vi "VI Reference Includes.vi"   [LabVIEW 2013, in "Engine Runtime Interface.lvclass"]
uses:
  Engine Runtime Interface.lvclass
  Engine Configuration/add and map fixed channel mapping.vi
  Engine Configuration/rename channel in mapping.vi
  Engine Configuration/apply mapping changes.vi
  Engine Configuration/delete mapping by channel.vi
  Engine Configuration/add mapping.vi
  Engine Configuration/apply tag changes.vi
  Engine Configuration/locate tag by name.vi
  Engine Configuration/delete tag.vi
  Engine Configuration/change tag metadata.vi
  Engine Configuration/change tag raw default value.vi
  Engine Configuration/change tag type.vi
  Engine Configuration/rename tag.vi
  Engine Configuration/add tag.vi
  Engine Configuration/Mappings.ctl
  Engine Configuration/Module Mappings.ctl
  Engine Configuration/Tag Info.ctl
  Engine Configuration/instance count allowed.vi
  Engine Configuration/get runtime class name.vi
  Engine Configuration/Get Supported Targets.vi
  Engine Configuration/filter tags by writer.vi
  Engine Configuration/filter tags by owner.vi
  Engine Configuration/filter tags by readers.vi
  Engine Configuration/filter tags available for mapping to channel.vi
  Engine Configuration/get full tag list.vi
  Engine Configuration/find tag mapped to channel.vi
  Engine Configuration/engine version.vi
  Engine Configuration/from string.vi
  Engine Configuration/to string.vi
  Engine Configuration/validate configuration.vi
  Get Unmapped Outputs.vi
  Get Mapping By Type.vi
  Find Tag From Channel Name.vi
  Find Components Mapping From Component or Channel Name.vi
  Create New Tags and Mappings.vi
  Append New Mappings.vi
  Create Tag Channel Pair.vi
  Execution States.ctl
  Open.vi
  Initialize.vi
  Start.vi
  Set Safe State.vi
  Pause.vi
  Get State.vi
  Stop.vi
  Close.vi
  Discover Channels.vi
  Engine Configuration/dynamic tag creation and mapping.vi
  Engine Configuration/engine configuration.lvclass
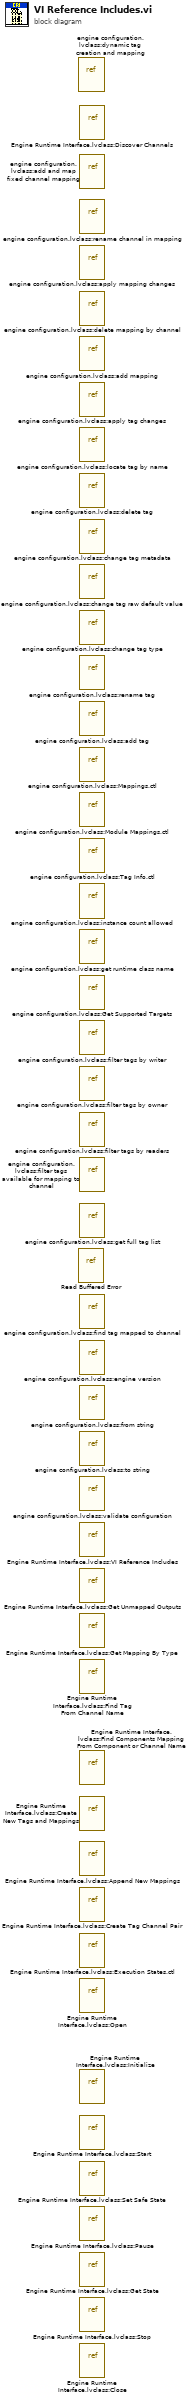
[diagram p0: block diagram]
diagram:
  n1 = vi-ref "Read Buffered Error.vi"() -> ()  [unwired: 1 out]
  n2 = vi-ref "engine configuration.lvclass:dynamic tag creation and mapping.vi"() -> ()  [unwired: 1 out]
  n3 = vi-ref "Engine Runtime Interface.lvclass:Discover Channels.vi"() -> ()  [unwired: 1 out]
  n4 = vi-ref "engine configuration.lvclass:add and map fixed channel mapping.vi"() -> ()  [unwired: 1 out]
  n5 = vi-ref "engine configuration.lvclass:rename channel in mapping.vi"() -> ()  [unwired: 1 out]
  n6 = vi-ref "engine configuration.lvclass:apply mapping changes.vi"() -> ()  [unwired: 1 out]
  n7 = vi-ref "engine configuration.lvclass:delete mapping by channel.vi"() -> ()  [unwired: 1 out]
  n8 = vi-ref "engine configuration.lvclass:add mapping.vi"() -> ()  [unwired: 1 out]
  n9 = vi-ref "engine configuration.lvclass:apply tag changes.vi"() -> ()  [unwired: 1 out]
  n10 = vi-ref "engine configuration.lvclass:locate tag by name.vi"() -> ()  [unwired: 1 out]
  n11 = vi-ref "engine configuration.lvclass:delete tag.vi"() -> ()  [unwired: 1 out]
  n12 = vi-ref "engine configuration.lvclass:change tag metadata.vi"() -> ()  [unwired: 1 out]
  n13 = vi-ref "engine configuration.lvclass:change tag raw default value.vi"() -> ()  [unwired: 1 out]
  n14 = vi-ref "engine configuration.lvclass:change tag type.vi"() -> ()  [unwired: 1 out]
  n15 = vi-ref "engine configuration.lvclass:rename tag.vi"() -> ()  [unwired: 1 out]
  n16 = vi-ref "engine configuration.lvclass:add tag.vi"() -> ()  [unwired: 1 out]
  n17 = vi-ref "engine configuration.lvclass:Mappings.ctl"() -> ()  [unwired: 1 out]
  n18 = vi-ref "engine configuration.lvclass:Module Mappings.ctl"() -> ()  [unwired: 1 out]
  n19 = vi-ref "engine configuration.lvclass:Tag Info.ctl"() -> ()  [unwired: 1 out]
  n20 = vi-ref "engine configuration.lvclass:instance count allowed.vi"() -> ()  [unwired: 1 out]
  n21 = vi-ref "engine configuration.lvclass:get runtime class name.vi"() -> ()  [unwired: 1 out]
  n22 = vi-ref "engine configuration.lvclass:Get Supported Targets.vi"() -> ()  [unwired: 1 out]
  n23 = vi-ref "engine configuration.lvclass:filter tags by writer.vi"() -> ()  [unwired: 1 out]
  n24 = vi-ref "engine configuration.lvclass:filter tags by owner.vi"() -> ()  [unwired: 1 out]
  n25 = vi-ref "engine configuration.lvclass:filter tags by readers.vi"() -> ()  [unwired: 1 out]
  n26 = vi-ref "engine configuration.lvclass:filter tags available for mapping to channel.vi"() -> ()  [unwired: 1 out]
  n27 = vi-ref "engine configuration.lvclass:get full tag list.vi"() -> ()  [unwired: 1 out]
  n28 = vi-ref "engine configuration.lvclass:find tag mapped to channel.vi"() -> ()  [unwired: 1 out]
  n29 = vi-ref "engine configuration.lvclass:engine version.vi"() -> ()  [unwired: 1 out]
  n30 = vi-ref "engine configuration.lvclass:from string.vi"() -> ()  [unwired: 1 out]
  n31 = vi-ref "engine configuration.lvclass:to string.vi"() -> ()  [unwired: 1 out]
  n32 = vi-ref "engine configuration.lvclass:validate configuration.vi"() -> ()  [unwired: 1 out]
  n33 = vi-ref "Engine Runtime Interface.lvclass:VI Reference Includes.vi"() -> ()  [unwired: 1 out]
  n34 = vi-ref "Engine Runtime Interface.lvclass:Get Unmapped Outputs.vi"() -> ()  [unwired: 1 out]
  n35 = vi-ref "Engine Runtime Interface.lvclass:Get Mapping By Type.vi"() -> ()  [unwired: 1 out]
  n36 = vi-ref "Engine Runtime Interface.lvclass:Find Tag From Channel Name.vi"() -> ()  [unwired: 1 out]
  n37 = vi-ref "Engine Runtime Interface.lvclass:Find Components Mapping From Component or Channel Name.vi"() -> ()  [unwired: 1 out]
  n38 = vi-ref "Engine Runtime Interface.lvclass:Create New Tags and Mappings.vi"() -> ()  [unwired: 1 out]
  n39 = vi-ref "Engine Runtime Interface.lvclass:Append New Mappings.vi"() -> ()  [unwired: 1 out]
  n40 = vi-ref "Engine Runtime Interface.lvclass:Create Tag Channel Pair.vi"() -> ()  [unwired: 1 out]
  n41 = vi-ref "Engine Runtime Interface.lvclass:Execution States.ctl"() -> ()  [unwired: 1 out]
  n42 = vi-ref "Engine Runtime Interface.lvclass:Open.vi"() -> ()  [unwired: 1 out]
  n43 = vi-ref "Engine Runtime Interface.lvclass:Initialize.vi"() -> ()  [unwired: 1 out]
  n44 = vi-ref "Engine Runtime Interface.lvclass:Start.vi"() -> ()  [unwired: 1 out]
  n45 = vi-ref "Engine Runtime Interface.lvclass:Set Safe State.vi"() -> ()  [unwired: 1 out]
  n46 = vi-ref "Engine Runtime Interface.lvclass:Pause.vi"() -> ()  [unwired: 1 out]
  n47 = vi-ref "Engine Runtime Interface.lvclass:Get State.vi"() -> ()  [unwired: 1 out]
  n48 = vi-ref "Engine Runtime Interface.lvclass:Stop.vi"() -> ()  [unwired: 1 out]
  n49 = vi-ref "Engine Runtime Interface.lvclass:Close.vi"() -> ()  [unwired: 1 out]
